vi "FIFO Core U64 - FPGA RAM.vi"(0 "input data":u64, 1 "reset":bool, 2 "fifo memory":refnum<k21>, 3 "fifo depth":u8(ring)=10 items=["4"=2, "8"=3, "16"=4, "32"=5, "64"=6, "128"=7, "256"=8, "512"=9, "1024"=10, "2048"=11, "4096"=12, "8192"=13, "16384"=14, "32768"=15, "65536"=16], 9 "input valid":bool, 12 "ready for output":bool=TRUE) -> (4 "output data":u64, 6 "state":T1, 10 "output valid":bool, 14 "ready for input":bool)   [LabVIEW 2011, in "FIFO.lvlib"]
uses:
  <instrlib>/RF-RIO/FIFO/FIFO/FPGA/FIFO.lvlib
  <instrlib>/RF-RIO/FIFO/FIFO/FPGA/Public/FIFO State.ctl
  <vilib>/rvi/DataTransferAndStorage/Container/Common/niFpgaContainerExecOnDevCompGetState.vi
  <vilib>/rvi/Memory/Memory_Emulation/niFpgaMemoryEmulationValidateCache.vi
  <vilib>/rvi/DataTransferAndStorage/Container/Common/niFpgaContainerGetUniqueNameForEmu.vi
  <vilib>/rvi/Memory/Memory_Emulation/nirvimemoryEmulationManagerCache_InsertValue.vi
  <vilib>/Utility/error.llb/Clear Errors.vi
  <vilib>/rvi/Memory/Memory_Emulation/nirvimemoryEmulationManagerCache_GetValue.vi
  <vilib>/rvi/Memory/Memory_Emulation/nirvimemoryEmulationManagerCache_SetValue.vi
  <vilib>/rvi/DataTransferAndStorage/Container/XNode/niFpgaContainer.xnode
  <vilib>/rvi/Memory/Memory_Emulation/niFpgaMemoryEmulationRefIn.vi
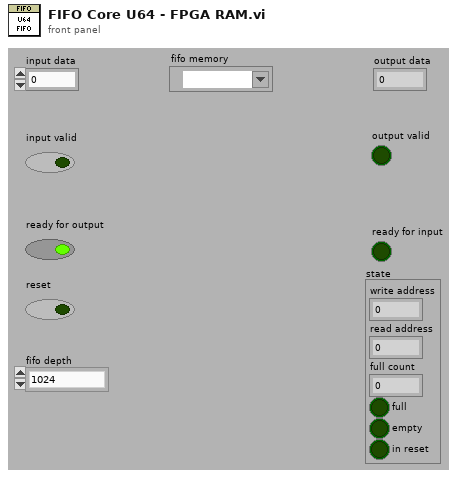
[diagram p1: front panel]
types:
  T1 = typedef "FIFO.lvlib/FIFO State.ctl" = cluster{"write address":u32, "read address":u32, "full count":u32, "full":bool, "empty":bool, "in reset":bool}
  T2 = typedef "FIFO.lvlib/FIFO State - 16-bit Address.ctl" = cluster{"write address":u16, "read address":u16, "full count":u16, "full":bool, "empty":bool}
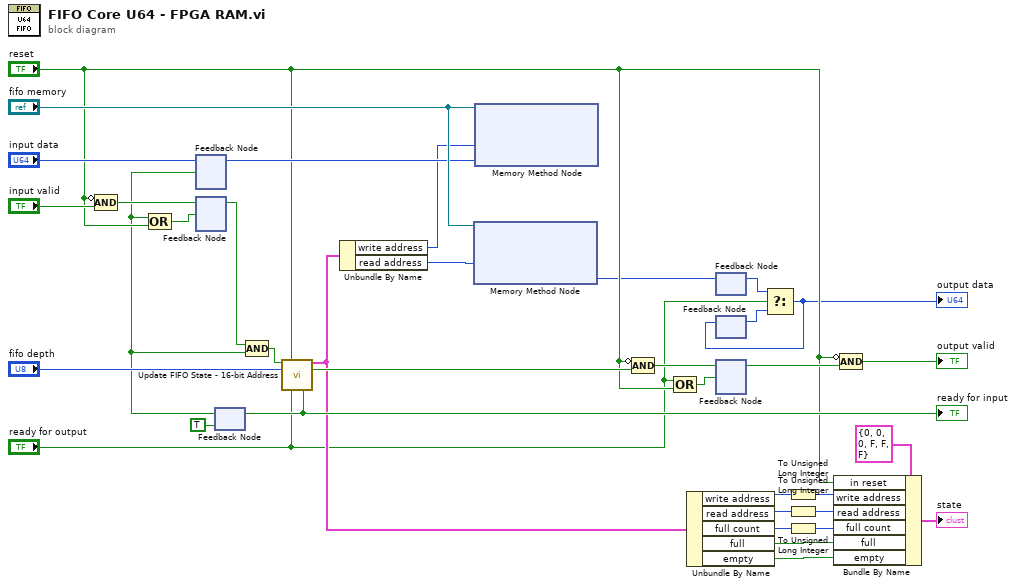
[diagram p0: block diagram]
diagram:
  n1 = Compound Arithmetic op=AND(invert "reset", "input valid") -> (w26:bool)
  n2 = feedback #1() -> (w30:u64)  [unwired: 1 in]
  n3 = feedback #2() -> (w9:bool)  [unwired: 1 in]
  n4 = feedback #3(TRUE ("ready for write")) -> (w8:bool)
  n5 = Compound Arithmetic op=OR(w8, "reset") -> (w25:bool)
  n6 = feedback-in #1("input data", w8) -> ()
  n7 = feedback-in #2(w26, w25) -> ()
  n8 = Compound Arithmetic op=AND(w9, w8) -> (w7:bool)
  n9 = call <instrlib>:"Update FIFO State - 16-bit Address.vi"("issue write"=w7, "reset"="reset", "fifo depth"="fifo depth", "ready for read request"="ready for output") -> ("state"=w10:T2, "issue read request"=w23:bool, "ready for write"=w22:bool)  [unwired: 9 in]
  "ready for input" <- w22
  n10 = feedback-in #3(w22) -> ()
  n11 = Unbundle By Name(w10) -> ("write address"=w29:u16, "read address"=w28:u16)
  n12 = xnode ("Memory Method Node")("Address"=w28, "Memory In"="fifo memory") -> ("Data"=w5:u64)  [unwired: 1 out]
  n13 = xnode ("Memory Method Node")("Address"=w29, "Data"=w30, "Memory In"="fifo memory") -> ()  [unwired: 1 out]
  n14 = Compound Arithmetic op=AND(invert "reset", w23) -> (w33:bool)
  n15 = Compound Arithmetic op=OR("ready for output", "reset") -> (w31:bool)
  n16 = Unbundle By Name(w10) -> ("write address"=w20:u16, "read address"=w19:u16, "full count"=w18:u16, "full"=w17:bool, "empty"=w16:bool)
  n17 = feedback #4() -> (w4:u64)  [unwired: 1 in]
  n18 = feedback-in #4(w5) -> ()
  n19 = feedback #5() -> (w3:u64)  [unwired: 1 in]
  n20 = feedback #6() -> (w32:bool)  [unwired: 1 in]
  n21 = feedback-in #6(w33, w31) -> ()
  n22 = Select(t=w4, s="ready for output", f=w3) -> (s? t:f=w1:u64)
  "output data" <- w1
  n23 = feedback-in #5(w1) -> ()
  n24 = To Unsigned Long Integer(number=w20) -> (unsigned 32bit integer=w13:u32)
  n25 = To Unsigned Long Integer(number=w19) -> (unsigned 32bit integer=w12:u32)
  n26 = To Unsigned Long Integer(number=w18) -> (unsigned 32bit integer=w11:u32)
  n27 = Bundle By Name(cluster=T1 {"write address"=0, "read address"=0, "full count"=0, "full"=FALSE, "empty"=FALSE, "in reset"=FALSE} ("state"), "in reset"="reset", "write address"=w13, "read address"=w12, "full count"=w11, "full"=w17, "empty"=w16) -> (→"state":T1)
  n28 = Compound Arithmetic op=AND(invert "reset", w32) -> (→"output valid":bool)
